vi "Host_Test.vi"() -> ()   [LabVIEW 2012]
uses:
  <vilib>/FPGAPlugInAG/PXIe-7962R/niLvFpga_Open_PXIe-7962R.vi
  <vilib>/rvi/interface/common/dynamic/niFpgaDynamicAddResources.vi
  <vilib>/Utility/error.llb/Error Cluster From Error Code.vi
  <vilib>/rvi/errors/niLvFpgaAdjustHostInterfaceError.vi
  <vilib>/FPGAPlugInAG/Dynamic/niLvFpga_Close_Dynamic.vi
  <vilib>/rvi/interface/nirviOpenFPGA/nirviOpenFPGA.xnode
  Scope/fpga_labview/FPGA Bitfiles/AnalogIntegrator_NI5771_PXIe-7962R.lvbitx
  FPGA VIs/AnalogIntegrator_NI5771_Resonance.vi
  <vilib>/rvi/interface/nirviReadWriteControl/nirviReadWriteControl.xnode
  <vilib>/rvi/interface/nirviMethod/nirviMethod.xnode
  <vilib>/rvi/interface/nirviCloseFPGA/nirviCloseFPGA.xnode
  <vilib>/rvi/interface/Simulation/niFpgaSimulationCallBeginRW.vi
  NiFpgaLv.dll
  <vilib>/FPGAPlugInAG/Dynamic/niLvFpga_ReadFifo_Dynamic.vi
  <vilib>/rvi/errors/niLvFpgaMergeErrorWithErrorCode.vi
panel:
  out "Resonance Trigger":u32[](graph)
  out "Samples per pixel":u32
  in  "Pixel time":dbl
  out "error out":errorcluster
  out "InterloopFIFO Overflow":bool
  out "ToHostCh1FIFO Overflow":bool
  out "Configured?":bool
  out "IO Module\\AI Over Range":bool
  out "Ch1":u32[](graph)
  # "microseconds"
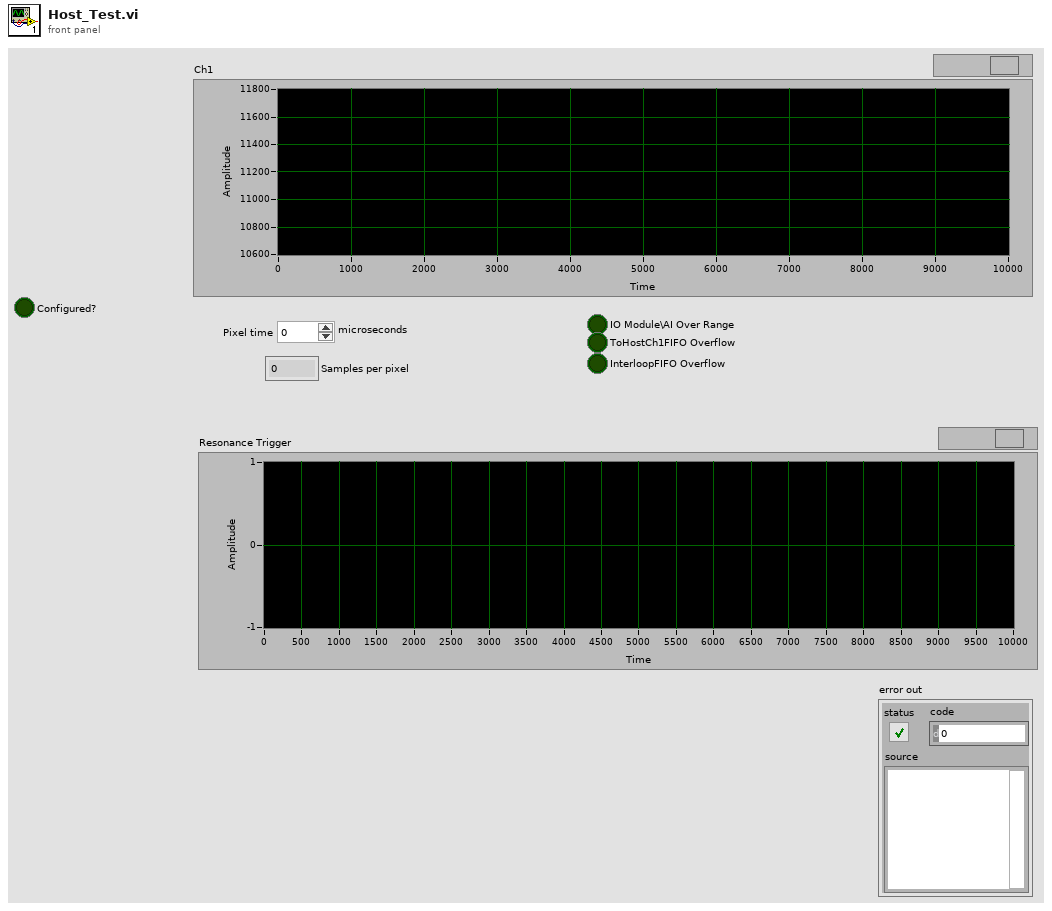
[diagram p1: front panel]
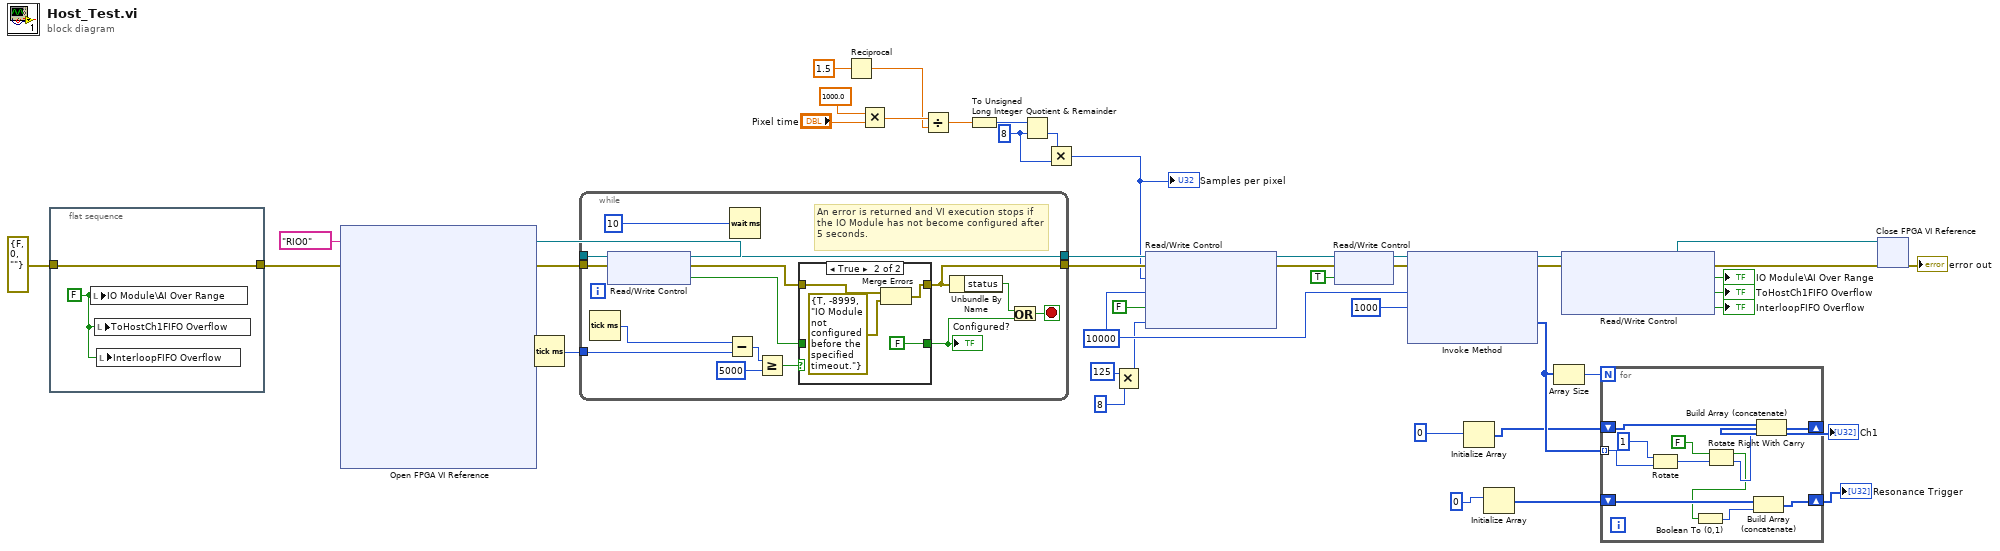
[diagram p0: block diagram]
diagram:
  w10 = u32 8 ("y")
  w37 = u32 10000 ("Requested pixels")
  n1 = flat-sequence {
    tunnel: errorcluster {"status"=FALSE, "code"=0, "source"=""} ("error in") -> [w46]
    tunnel: [w46] -> w20
    frame #0 {
      w47 = FALSE ("IO Module\\AI Over Range")
      n2 = local write "IO Module\\AI Over Range"(w47) -> ()
      n3 = local write "ToHostCh1FIFO Overflow"(w47) -> ()
      n4 = local write "InterloopFIFO Overflow"(w47) -> ()
    }
  }
  n5 = xnode "Open FPGA VI Reference"("error in"=w20, "resource name"=tag "RIO0") -> ("FPGA VI Reference Out"=w30:refnum<k20>, "error out"=w31:errorcluster)
  n6 = Tick Count (ms)() -> (millisecond timer value=w29:u32)
  n7 = while {
    tunnel: w31 -> [w55]
    tunnel: [w59] -> w28
    tunnel: [w51] -> w27
    tunnel: w30 -> [w54]
    tunnel: w29 -> [w49]
    stop <- w57 stop-if-true
    # "An error is returned and VI execution stops if the IO Module has not become configured after 5 seconds."
    n8 = Tick Count (ms)() -> (millisecond timer value=w50:u32)
    n9 = xnode "Read/Write Control"("FPGA VI Reference In"=w54, "error in"=w55) -> ("FPGA VI Reference Out"=w51:refnum<k20>, "error out"=w52:errorcluster, "Configured?"=w53:bool)
    n10 = Subtract(x=w50, y=w49) -> (x-y=w48:u32)
    n11 = Wait (ms)(milliseconds to wait=u32 10) -> ()  [unwired: 1 out]
    n12 = Greater Or Equal?(x=w48, y=u32 5000) -> (x >= y?=w60:bool)
    n13 = case shown="True" w60 {
      tunnel: [w64 FALSE ("Configured?")] -> w56
      tunnel: w53 -> [w64 _]
      tunnel: [w63 w67] -> w59
      tunnel: w52 -> [w63 w65]
      frame False {
      }
      frame True {
        n14 = Merge Errors(w65, errorcluster {"status"=TRUE, "code"=-8999, "source"="IO Module not configured before the specified timeout."} ("error in")) -> (w67:errorcluster)
      }
    }
    "Configured?" <- w56
    n15 = Unbundle By Name(w59) -> ("status"=w58:bool)
    n16 = Or(x=w58, y=w56) -> (x .or. y?=w57:bool)
  }
  n17 = Reciprocal(x=1.5) -> (1/x=w14:dbl)
  n18 = Multiply(x=1000.0, y="Pixel time") -> (x*y=w15:dbl)
  n19 = Divide(x=w15, y=w14) -> (x/y=w13:dbl)
  n20 = To Unsigned Long Integer(number=w13) -> (unsigned 32bit integer=w12:u32)
  n21 = Quotient & Remainder(x=w12, y=w10) -> (floor(x/y)=w11:u32)  [unwired: 1 out]
  n22 = Multiply(x=w11, y=w10) -> (x*y=w9:u32)
  "Samples per pixel" <- w9
  n23 = Multiply(x=125, y=8) -> (x*y=w24:i32)
  n24 = xnode "Read/Write Control"("FPGA VI Reference In"=w27, "error in"=w28, "Samples per pixel"=w9, "Requested pixels"=w37, "Acquire continuously"=FALSE, "Baselinex8 Ch1"=w24) -> ("FPGA VI Reference Out"=w42:refnum<k20>, "error out"=w43:errorcluster)
  n25 = xnode "Read/Write Control"("FPGA VI Reference In"=w42, "error in"=w43, "Acquire"=TRUE) -> ("FPGA VI Reference Out"=w40:refnum<k20>, "error out"=w39:errorcluster)
  n26 = xnode "Invoke Method"("FPGA VI Reference In"=w40, "error in"=w39, "Number of Elements"=w37, "Timeout (ms)"=1000) -> ("FPGA VI Reference Out"=w36:refnum<k20>, "error out"=w34:errorcluster, "Data"=w8:u32[])  [unwired: 1 out]
  n27 = Initialize Array(u32 0) -> (w5:u32[])  [unwired: 1 in]
  n28 = Initialize Array(u32 0) -> (w2:u32[])  [unwired: 1 in]
  n29 = Array Size(array=w8) -> (size(s)=w7:i32)
  n30 = xnode "Read/Write Control"("FPGA VI Reference In"=w36, "error in"=w34) -> ("FPGA VI Reference Out"=w35:refnum<k20>, "error out"=w33:errorcluster, "IO Module\\AI Over Range"=→"IO Module\\AI Over Range":bool, "ToHostCh1FIFO Overflow"=→"ToHostCh1FIFO Overflow":bool, "InterloopFIFO Overflow"=→"InterloopFIFO Overflow":bool)
  n31 = for {
    N: w7 -> [_]
    tunnel: w8 -> [w69] mode=indexing
    shift-right: [w78] -> w4
    shift-left: w5 -> [w79]
    shift-right: [w77] -> w1
    shift-left: w2 -> [w76]
    n32 = Rotate(1:w69, 2:1) -> (0:w74:u32)
    n33 = Rotate Right With Carry(2:w74, 3:FALSE) -> (0:w72:u32, 1:w71:bool)
    n34 = Boolean To (0,1)(Boolean=w71) -> (0, 1=w70:i16)
    n35 = Build Array (concatenate)(w76, w70) -> (w77:u32[])
    n36 = Build Array (concatenate)(w79, w72) -> (w78:u32[])
  }
  "Ch1" <- w4
  "Resonance Trigger" <- w1
  n37 = xnode "Close FPGA VI Reference"("FPGA VI Reference In"=w35, "error in"=w33) -> ("error out"=→"error out":errorcluster)
